vi "Read Speed.vi"(8 "error in (no error)":errorcluster, 11 "Iterative Dispense in":refnum<class "Baseplate Dispense.lvclass">) -> (0 "error out":errorcluster, 2 "Speed":dbl, 3 "Iterative Dispense out":refnum<class "Baseplate Dispense.lvclass">)   [LabVIEW 2016, in "Baseplate Dispense.lvclass"]
uses:
  Baseplate Dispense.lvclass
  Baseplate Dispense.lvclass/Baseplate Dispense.ctl
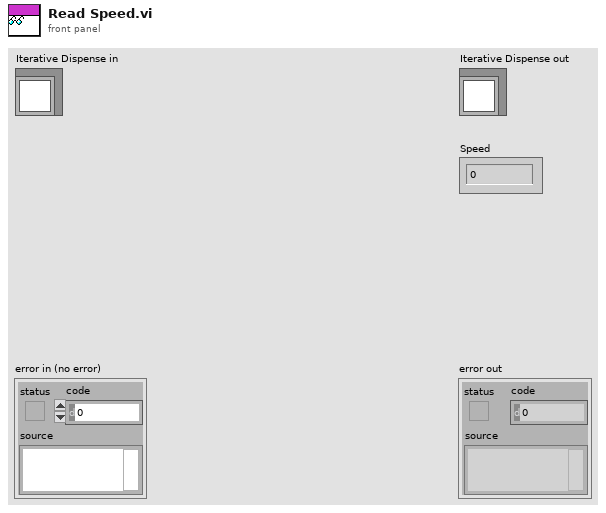
[diagram p1: front panel]
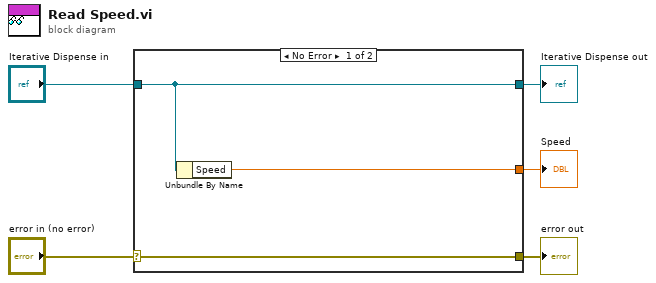
[diagram p0: block diagram]
diagram:
  n1 = case shown="No Error" "error in (no error)" {
    selector: "error in (no error)" -> [w8 w9]
    tunnel: [w8 w9] -> w4
    tunnel: [w7 w10] -> w2
    tunnel: "Iterative Dispense in" -> [w7 w10]
    tunnel: [w6 _] -> w1
    frame No Error {
      n2 = Unbundle By Name(w7) -> ("Speed"=w6:dbl)
    }
    frame Error {
    }
  }
  "error out" <- w4
  "Iterative Dispense out" <- w2
  "Speed" <- w1
